vi "New Pulse Acquired.vi"(8 "error in (no error)":errorcluster, 10 "Result in":refnum<class "Acquired Result.lvclass">, 11 "Monitor-Pulse in":refnum<class "Monitor-Pulse.lvclass">) -> (0 "error out":errorcluster, 3 "Monitor-Pulse out":refnum<class "Monitor-Pulse.lvclass">)   [LabVIEW 2016, in "Monitor-Pulse.lvclass"]
uses:
  Monitor-Pulse.lvclass
  Results/Acquired Result/Acquired Result.lvclass
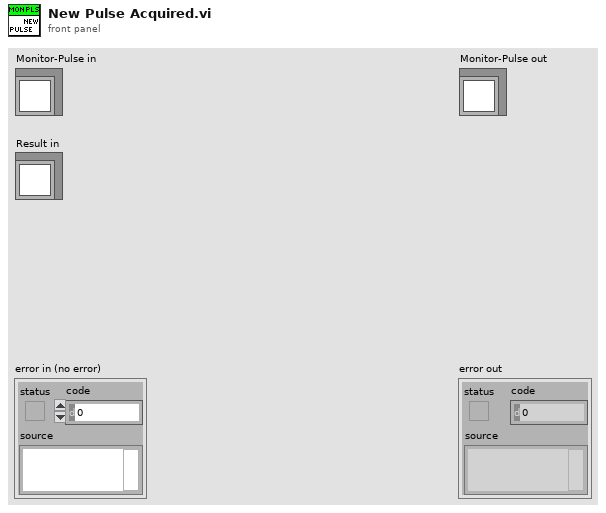
[diagram p1: front panel]
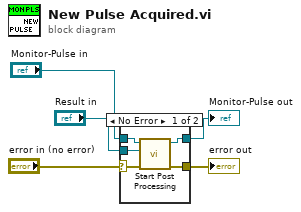
[diagram p0: block diagram]
diagram:
  n1 = case shown="No Error" "error in (no error)" {
    selector: "error in (no error)" -> [w10 w12]
    tunnel: [w6 w12] -> w4
    tunnel: [w7 w11] -> w2
    tunnel: "Monitor-Pulse in" -> [w9 w11]
    tunnel: "Result in" -> [w8 _]
    frame No Error {
      n2 = call-dynamic "Start Post Processing.vi"("error in (no error)"=w10, "Result in"=w8, "Monitor-Pulse in"=w9) -> ("error out"=w6:errorcluster, "Monitor-Pulse out"=w7:refnum<class "Monitor-Pulse.lvclass">)  [unwired: 7 in]
    }
    frame Error {
    }
  }
  "error out" <- w4
  "Monitor-Pulse out" <- w2
